vi "createSharedEvnts.vi"(8 "error in (no error)":errorcluster, 11 "SAL_Events in":refnum<class "SAL_Events.lvclass">) -> (0 "error out":errorcluster, 3 "SAL_Events out":refnum<class "SAL_Events.lvclass">)   [LabVIEW 2016, in "SAL_Events.lvclass"]
uses:
  SAL_Events.lvclass
  sharedEvents.ctl
  SAL_Events.lvclass/SAL_Events.ctl
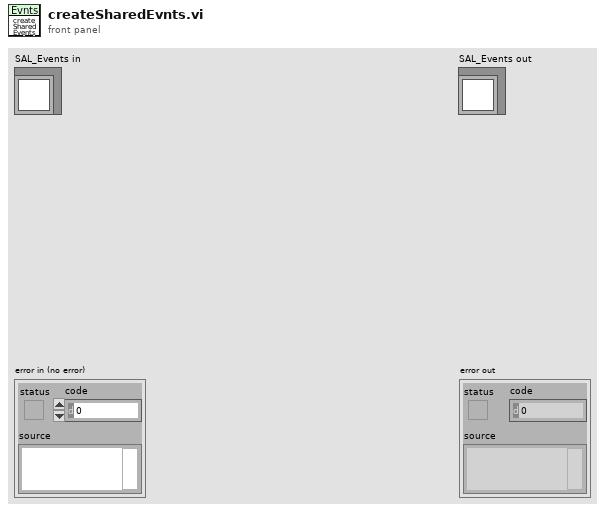
[diagram p1: front panel]
types:
  T1 = typedef "sharedEvents.ctl" = cluster{"stopApp":refnum<user-event>}
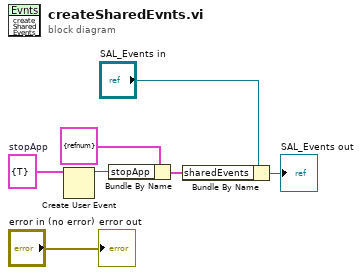
[diagram p0: block diagram]
diagram:
  w3 = cluster{"stop":bool} {"stop"=TRUE}  # stopApp
  n1 = Create User Event(user event datatype=w3) -> (user event=w1:refnum<user-event>)  [unwired: 1 in, 1 out]
  n2 = Bundle By Name(cluster=T1 {"stopApp"=refnum} ("sharedEvents"), "stopApp"=w1) -> (w4:T1)
  n3 = Bundle By Name(cluster="SAL_Events in", "sharedEvents"=w4) -> (→"SAL_Events out":refnum<class "SAL_Events.lvclass">)
  "error out" <- "error in (no error)"
